vi "Write log to file.vi"(4 "prefix":string, 5 "version":string, 6 "current priority":string, 7 "enabled priority":string, 8 "error in":errorcluster, 9 "resp array":string[](array[string]), 10 "send array":string[](array[string])) -> (0 "error out":errorcluster, 1 "error":bool, 2 "logged text":string)   [LabVIEW 2018]
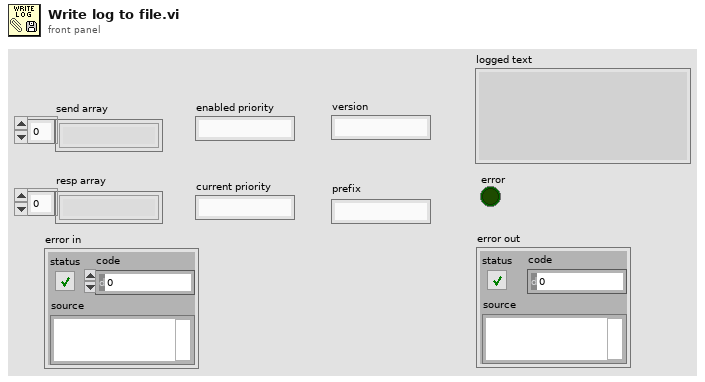
[diagram p1: front panel]
types:
  T1 = enum16{"open", "replace", "create", "open or create", "replace or create", "replace or create with confirmation"}
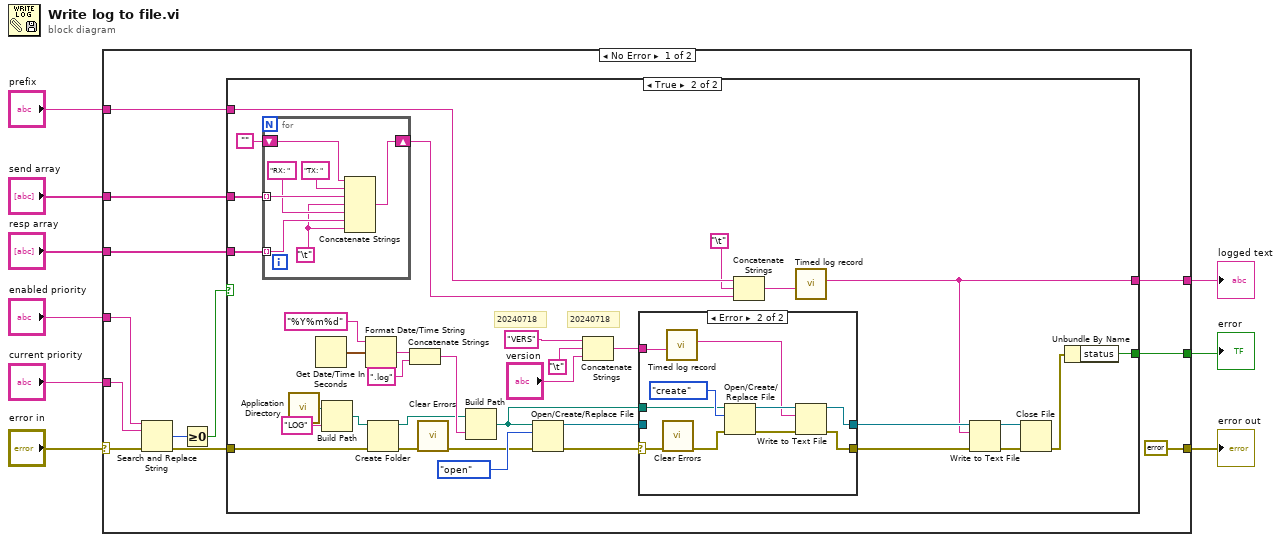
[diagram p0: block diagram]
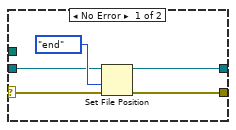
[diagram p3: hidden frame]
diagram:
  n1 = case shown="No Error" "error in" {
    selector: "error in" -> [w14 _]
    tunnel: "enabled priority" -> [w15 _]
    tunnel: [errorcluster {"status"=FALSE, "code"=0, "source"=""} ("error out") _] -> w8
    tunnel: [w21 _] -> w6
    tunnel: "current priority" -> [w12 _]
    tunnel: "resp array" -> [w19 _]
    tunnel: "send array" -> [w18 _]
    tunnel: "prefix" -> [w16 _]
    tunnel: [w17 _] -> w1
    frame No Error {
      n2 = Search and Replace String(input string=w15, search string=w12, error in=w14) -> (number of replacements=w11:i32, error out=w13:errorcluster)  [unwired: 5 in, 2 out]
      n3 = Greater Or Equal To 0?(x=w11) -> (x >= 0?=w10:bool)
      n4 = case shown="True" w10 {
        tunnel: [_ w55] -> w21
        tunnel: w19 -> [_ w54]
        tunnel: w18 -> [_ w53]
        tunnel: [_ w22] -> w17
        tunnel: w16 -> [_ w35]
        tunnel: w13 -> [_ w51]
        frame False {
        }
        frame True {
          # "20240718"
          # "20240718"
          n5 = for {
            tunnel: w54 -> [w75] mode=indexing
            tunnel: w53 -> [w77] mode=indexing
            shift-right: [w72] -> w33
            shift-left: "" -> [w73]
            w71 = "\t"
            n6 = Concatenate Strings(w73, "TX: ", w77, w71, "RX: ", w75, w71) -> (w72:string)
          }
          n7 = call <vilib>:"Application Directory.vi"() -> ("Application Directory"=w50:path)
          n8 = Get Date/Time In Seconds() -> (seconds since 1Jan1904=w48:timestamp)
          n9 = Build Path(base path=w50, name or relative path="LOG") -> (appended path=w40:path)
          n10 = Format Date/Time String(time format string (%c)="%Y%m%d", seconds (now)=w48) -> (date/time string=w46:string)  [unwired: 1 in]
          n11 = Create Folder(path (use dialog)=w40, error in=w51) -> (created path=w37:path, error out=w39:errorcluster)  [unwired: 1 in, 1 out]
          n12 = Concatenate Strings(w46, ".log" ("string")) -> (w45:string)
          n13 = call <vilib>:"Clear Errors.vi"("error in (no error)"=w39) -> ("error out"=w38:errorcluster)  [unwired: 5 in, 1 out]
          n14 = Build Path(base path=w37, name or relative path=w45) -> (appended path=w28:path)
          n15 = Open/Create/Replace File(file path (use dialog)=w28, error in=w38, operation (0:open)=T1."open") -> (refnum out=w31:refnum<file>, error out=w32:errorcluster)  [unwired: 3 in, 1 out]
          n16 = Concatenate Strings("VERS" ("string"), "\t", "version") -> (w27:string)
          n17 = case shown="Error" w32 {
            selector: w32 -> [w59 w70]
            tunnel: w31 -> [w58 _]
            tunnel: [w57 w63] -> w30
            tunnel: [w56 w64] -> w29
            tunnel: w28 -> [_ w68]
            tunnel: w27 -> [_ w62]
            frame No Error {
              n18 = Set File Position(refnum=w58, from (0:start)=enum16{"start", "end", "current"}."end", error in=w59) -> (refnum out=w57:refnum<file>, error out=w56:errorcluster)  [unwired: 1 in]
            }
            frame Error {
              n19 = call <vilib>:"Clear Errors.vi"("error in (no error)"=w70) -> ("error out"=w67:errorcluster)  [unwired: 5 in, 1 out]
              n20 = call "Timed log record .vi"("log input"=w62) -> ("log register"=w61:string)  [unwired: 9 in, 1 out]
              n21 = Open/Create/Replace File(file path (use dialog)=w68, error in=w67, operation (0:open)=T1."create") -> (refnum out=w65:refnum<file>, error out=w66:errorcluster)  [unwired: 3 in, 1 out]
              n22 = Write to Text File(file (use dialog)=w65, text=w61, error in=w66) -> (refnum out=w63:refnum<file>, error out=w64:errorcluster)  [unwired: 1 in, 1 out]
            }
          }
          n23 = Concatenate Strings(w35, "\t", w33) -> (w23:string)
          n24 = call "Timed log record .vi"("log input"=w23) -> ("log register"=w22:string)  [unwired: 9 in, 1 out]
          n25 = Write to Text File(file (use dialog)=w30, text=w22, error in=w29) -> (refnum out=w43:refnum<file>, error out=w42:errorcluster)  [unwired: 1 in, 1 out]
          n26 = Close File(refnum=w43, error in=w42) -> (error out=w41:errorcluster)  [unwired: 1 out]
          n27 = Unbundle By Name(w41) -> ("status"=w55:bool)
        }
      }
    }
    frame Error {
    }
  }
  "error out" <- w8
  "error" <- w6
  "logged text" <- w1
